vi "WLAN_FrameAnalysis_BothMessages - Optimized - Kopie_TDMA.vi"(8 "error in (no error)":errorcluster, 11 "input cluster":cluster{"t0":dbl, "dt":dbl, "Y":cdb[]}) -> (0 "error out":errorcluster, 1 "Constellation":cdb[](graph), 2 "Modulation parameter":T1, 3 "SC Bits":i8[](array[numeric]), 4 "Frequency offset":dbl, 5 "SIG valid?":bool, 7 "Base Bits":i8[](array[numeric]))   [LabVIEW 2022 SP3]
panel:
  out "x+y":dbl
  out "Frequency offset(LTF)":dbl
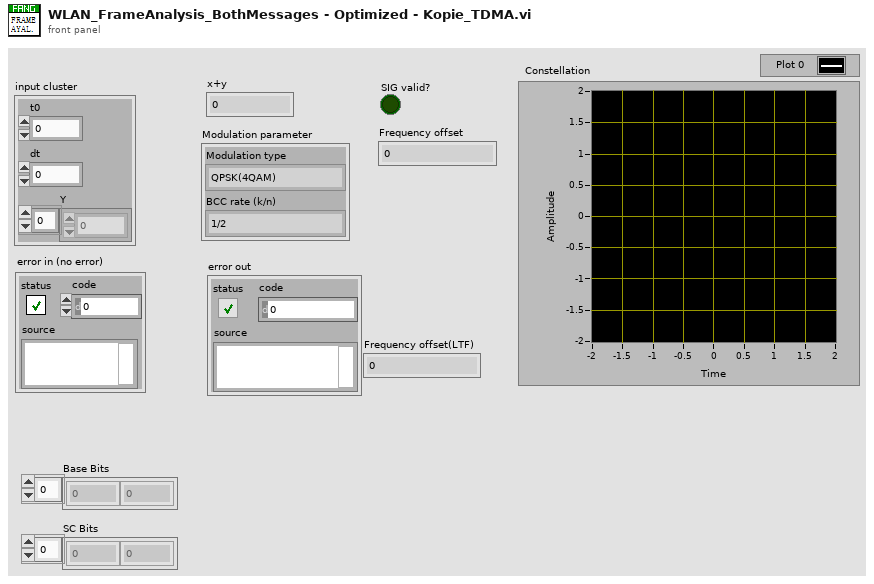
[diagram p1: front panel]
types:
  T1 = cluster{"Modulation type":enum16{"QPSK(4QAM)", "64QAM", "16QAM", "BPSK"}, "BCC rate (k/n)":enum16{"1/2", "2/3", "3/4"}}
  T2 = cluster{"Modulation type":enum16{"QPSK(4QAM)", "64QAM", "16QAM", "BPSK", "BPSK Vertical"}, "BCC rate (k/n)":enum16{"1/2", "2/3", "3/4"}}
  T3 = enum16{"QPSK(4QAM)", "64QAM", "16QAM", "BPSK", "BPSK Vertical"}
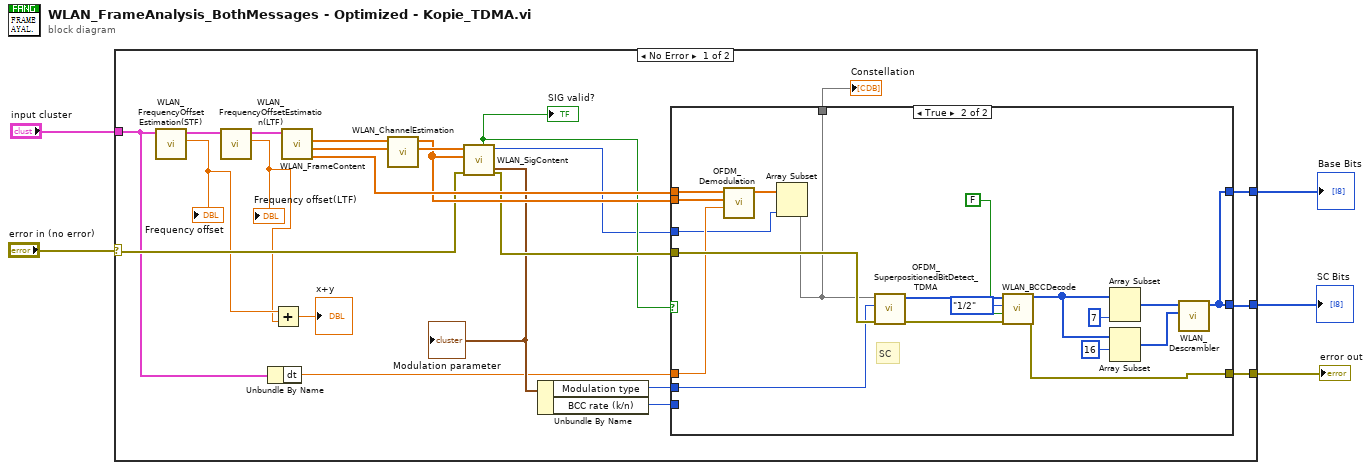
[diagram p0: block diagram]
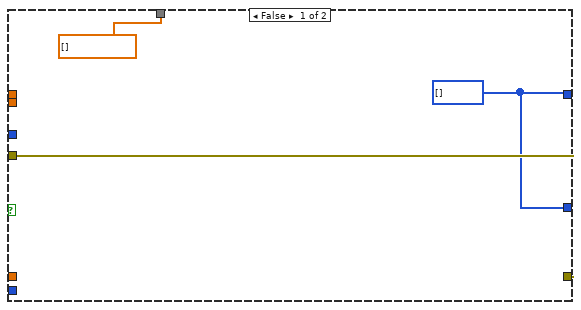
[diagram p2: hidden frame]
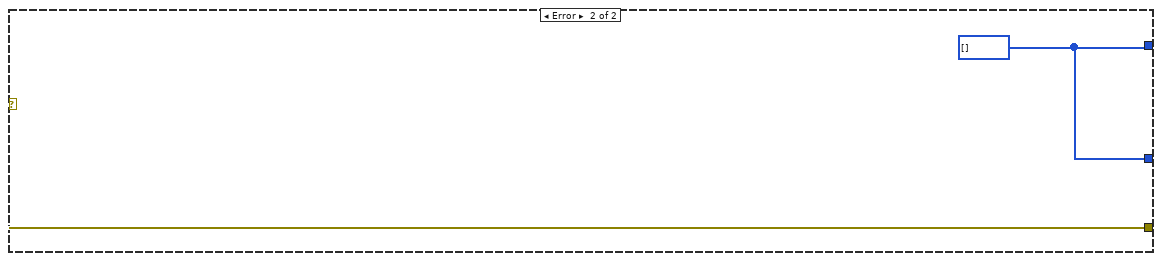
[diagram p3: hidden frame]
diagram:
  n1 = case shown="No Error" "error in (no error)" {
    selector: "error in (no error)" -> [w15 w51]
    tunnel: "input cluster" -> [w9 _]
    tunnel: [w22 w51] -> w4
    tunnel: [w21 w50] -> w3
    tunnel: [w7 w50] -> w1
    frame No Error {
      n2 = call "WLAN_FrequencyOffsetEstimation(STF).vi"("output cluster"=w9) -> ("Frequency offset(STF)"=w13:dbl, "output cluster 2"=w14:cluster{"t0":dbl, "dt":dbl, "Y":cdb[]})  [unwired: 8 in]
      "Frequency offset" <- w13
      n3 = call "WLAN_FrequencyOffsetEstimation(LTF).vi"("input cluster"=w14) -> ("Frequency offset(LTF)"=w12:dbl, "output cluster"=w10:cluster{"t0":dbl, "dt":dbl, "Y":cdb[]})  [unwired: 9 in]
      "Frequency offset(LTF)" <- w12
      n4 = Unbundle By Name(w9) -> ("dt"=w8:dbl)
      n5 = Add(x=w13, y=w12) -> (x+y=→"x+y":dbl)
      n6 = call "WLAN_FrameContent.vi"("Input cluster"=w10) -> ("DATA"=w27:cdb[], "SIG"=w25:cdb[], "LTF"=w26:cdb[])  [unwired: 7 in, 1 out]
      n7 = call "WLAN_ChannelEstimation.vi"("LTF"=w26) -> ("Frequency estimation"=w24:cdb[])  [unwired: 10 in]
      n8 = call "WLAN_SigContent.vi"("error in (no error)"=w15, "Frequency channel estimation"=w24, "SIG"=w25) -> ("error out"=w23:errorcluster, "original bit numbers"=w6:u32, "Modulation parameter"=w20:T2, "SIG valid?"=w16:bool)  [unwired: 3 in, 2 out]
      "Modulation parameter" <- w20
      "SIG valid?" <- w16
      n9 = Unbundle By Name(w20) -> ("Modulation type"=w19:T3, "BCC rate (k/n)"=w18:enum16{"1/2", "2/3", "3/4"})
      n10 = case shown="True" w16 {
        tunnel: w27 -> [_ w49]
        tunnel: [w30 w34] -> w22
        tunnel: w24 -> [_ w47]
        tunnel: w23 -> [w30 w46]
        tunnel: w6 -> [_ w31]
        tunnel: w19 -> [_ w45]
        tunnel: [w28 w33] -> w21
        tunnel: w18 -> [_ _]
        tunnel: [cdb[] [] w40] -> w17
        tunnel: w8 -> [_ w37]
        tunnel: [w28 w33] -> w7
        frame False {
          w28 = i8[] [] ("scrambled bits")
        }
        frame True {
          # "SC"
          n11 = call "OFDM_Demodulation.vi"("sampling period"=w37, "Frequency channel estimation"=w47, "Input sequence"=w49) -> ("Output sequence"=w48:cdb[])  [unwired: 7 in, 1 out]
          n12 = Array Subset(array=w48, length=w31) -> (w40:cdb[])  [unwired: 1 in]
          n13 = call "OFDM_SuperpositionedBitDetect_TDMA.vi"("Input symbols"=w40, "Modulation type"=w45, "error in (no error)"=w46) -> ("SC Bits"=w39:i8[], "error out"=w35:errorcluster)  [unwired: 4 in, 2 out]
          n14 = call "WLAN_BCCDecode.vi"("error in (no error)"=w35, "need add zeros?"=FALSE, "BCC rate (k/n)"=enum16{"1/2", "2/3", "3/4"}."1/2", "input bit stream"=w39) -> ("error out"=w34:errorcluster, "output bit stream"=w38:i8[])  [unwired: 6 in]
          n15 = Array Subset(array=w38, length=7) -> (w41:i8[])  [unwired: 1 in]
          n16 = Array Subset(array=w38, index=16) -> (w42:i8[])  [unwired: 1 in]
          n17 = call "WLAN_Descrambler.vi"("scrambler initial bits"=w41, "data bits"=w42) -> ("scrambled bits"=w33:i8[])  [unwired: 7 in]
        }
      }
      "Constellation" <- w17
    }
    frame Error {
      w50 = i8[] [] ("scrambled bits")
    }
  }
  "error out" <- w4
  "SC Bits" <- w3
  "Base Bits" <- w1
